vi "butterfly_valve_subvi.vi"(6 "Desired pressure":dbl, 8 "error in (no error)":errorcluster, 9 "Pressure Control":u32, 10 "?":dbl=100.0 min=0.0 max=100.0 step=5.0, 11 "VISA Refnum in":refnum<visa-resource-name>) -> (0 "error out":errorcluster, 2 "Valve position (%)":dbl, 3 "VISA Refnum out":refnum<visa-resource-name>)   [LabVIEW 2014]
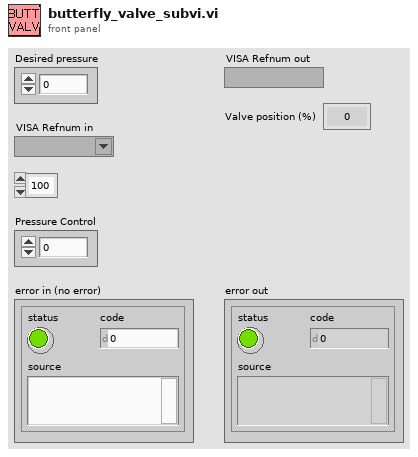
[diagram p1: front panel]
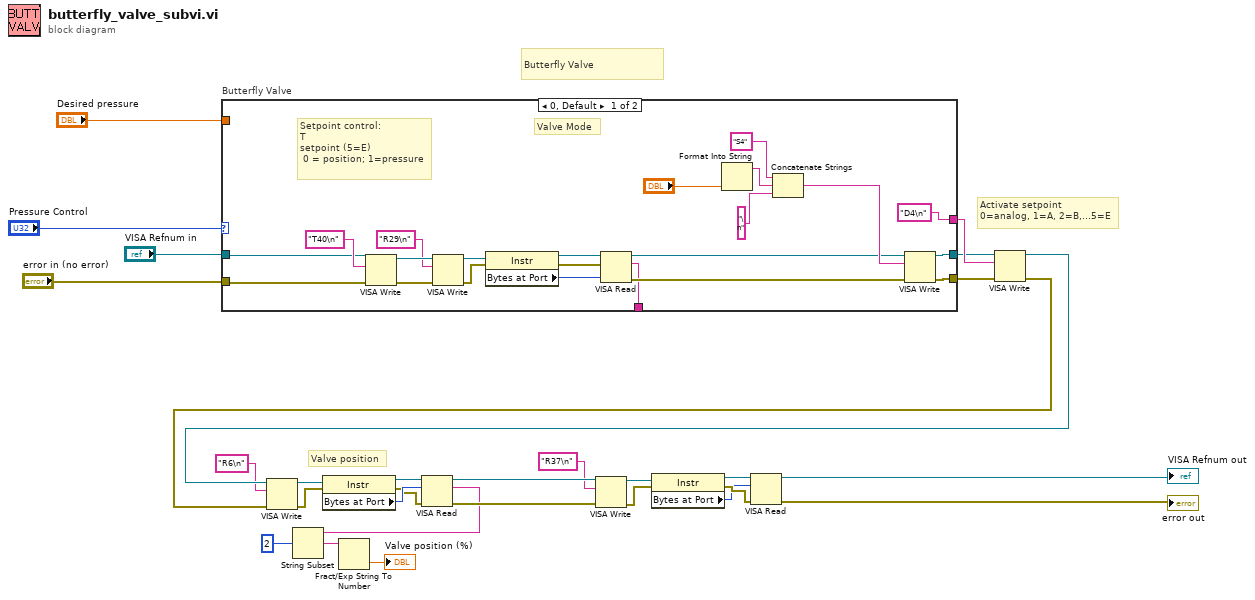
[diagram p0: block diagram]
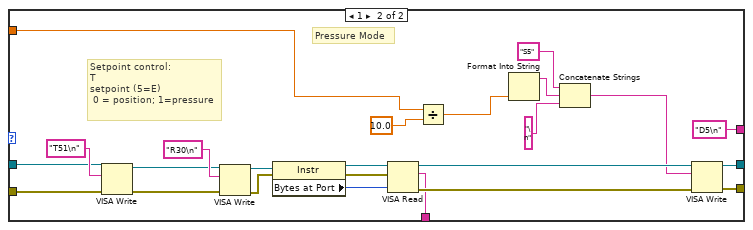
[diagram p2: hidden frame]
diagram:
  # "Activate setpoint \n0=analog, 1=A, 2=B,...5=E"
  # "Valve position"
  # "Butterfly Valve"
  n1 = case "Butterfly Valve" shown="0, Default" "Pressure Control" {
    tunnel: "VISA Refnum in" -> [w35 w57]
    tunnel: "error in (no error)" -> [w34 w58]
    tunnel: [w33 w60] -> w19
    tunnel: [w32 w59] -> w20
    tunnel: [w31 w56] -> _
    tunnel: ["D4\n" ("write buffer") "D5\n" ("write buffer")] -> w21
    tunnel: "Desired pressure" -> [_ w53]
    frame 0, Default {
      # "Valve Mode"
      # "Setpoint control:\nT\nsetpoint (5=E)\n 0 = position; 1=pressure"
      n2 = VISA Write(VISA resource name=w35, write buffer="T40\n", error in (no error)=w34) -> (VISA resource name out=w46:refnum<visa-resource-name>, error out=w44:errorcluster)  [unwired: 1 out]
      n3 = VISA Write(VISA resource name=w46, write buffer="R29\n", error in (no error)=w44) -> (VISA resource name out=w39:refnum<visa-resource-name>, error out=w40:errorcluster)  [unwired: 1 out]
      n4 = property class="Instr"(reference=w39, error in=w40) -> (reference out=w37:refnum<visa-resource-name>, error out=w38:errorcluster, "Bytes at Port"=w45:u32)
      n5 = VISA Read(VISA resource name=w37, byte count=w45, error in (no error)=w38) -> (VISA resource name out=w43:refnum<visa-resource-name>, read buffer=w31:string, error out=w42:errorcluster)  [unwired: 1 out]
      n6 = Format Into String("?") -> (resulting string=w51:string)  [unwired: 3 in, 1 out]
      n7 = Concatenate Strings("S4" ("string"), w51, "\n" ("string")) -> (w48:string)
      n8 = VISA Write(VISA resource name=w43, write buffer=w48, error in (no error)=w42) -> (VISA resource name out=w33:refnum<visa-resource-name>, error out=w32:errorcluster)  [unwired: 1 out]
    }
    frame 1 {
      # "Pressure Mode"
      # "Setpoint control:\nT\nsetpoint (5=E)\n 0 = position; 1=pressure"
      n9 = VISA Write(VISA resource name=w57, write buffer="T51\n", error in (no error)=w58) -> (VISA resource name out=w65:refnum<visa-resource-name>, error out=w67:errorcluster)  [unwired: 1 out]
      n10 = VISA Write(VISA resource name=w65, write buffer="R30\n", error in (no error)=w67) -> (VISA resource name out=w72:refnum<visa-resource-name>, error out=w71:errorcluster)  [unwired: 1 out]
      n11 = property class="Instr"(reference=w72, error in=w71) -> (reference out=w74:refnum<visa-resource-name>, error out=w73:errorcluster, "Bytes at Port"=w66:u32)
      n12 = VISA Read(VISA resource name=w74, byte count=w66, error in (no error)=w73) -> (VISA resource name out=w68:refnum<visa-resource-name>, read buffer=w56:string, error out=w69:errorcluster)  [unwired: 1 out]
      n13 = Divide(x=w53, y=10.0) -> (x/y=w52:dbl)
      n14 = Format Into String(w52) -> (resulting string=w61:string)  [unwired: 3 in, 1 out]
      n15 = Concatenate Strings("S5" ("string"), w61, "\n" ("string")) -> (w63:string)
      n16 = VISA Write(VISA resource name=w68, write buffer=w63, error in (no error)=w69) -> (VISA resource name out=w60:refnum<visa-resource-name>, error out=w59:errorcluster)  [unwired: 1 out]
    }
  }
  n17 = VISA Write(VISA resource name=w19, write buffer=w21, error in (no error)=w20) -> (VISA resource name out=w23:refnum<visa-resource-name>, error out=w24:errorcluster)  [unwired: 1 out]
  n18 = VISA Write(VISA resource name=w23, write buffer="R6\n", error in (no error)=w24) -> (VISA resource name out=w5:refnum<visa-resource-name>, error out=w6:errorcluster)  [unwired: 1 out]
  n19 = property class="Instr"(reference=w5, error in=w6) -> (reference out=w2:refnum<visa-resource-name>, error out=w3:errorcluster, "Bytes at Port"=w4:u32)
  n20 = VISA Read(VISA resource name=w2, byte count=w4, error in (no error)=w3) -> (VISA resource name out=w16:refnum<visa-resource-name>, read buffer=w7:string, error out=w17:errorcluster)  [unwired: 1 out]
  n21 = String Subset(string=w7, offset (0)=2) -> (substring=w9:string)  [unwired: 1 in]
  n22 = Fract/Exp String To Number(string=w9) -> (number=→"Valve position (%)":dbl)  [unwired: 3 in, 1 out]
  n23 = VISA Write(VISA resource name=w16, write buffer="R37\n", error in (no error)=w17) -> (VISA resource name out=w11:refnum<visa-resource-name>, error out=w10:errorcluster)  [unwired: 1 out]
  n24 = property class="Instr"(reference=w11, error in=w10) -> (reference out=w14:refnum<visa-resource-name>, error out=w13:errorcluster, "Bytes at Port"=w12:u32)
  n25 = VISA Read(VISA resource name=w14, byte count=w12, error in (no error)=w13) -> (VISA resource name out=→"VISA Refnum out":refnum<visa-resource-name>, error out=→"error out":errorcluster)  [unwired: 2 out]
